vi "Variant-to-String.vi"(11 "Cluster":cluster{"Name":string, "Variant Data":variant}) -> (0 "error out":errorcluster, 3 "String":string)   [LabVIEW 2016, in "SaveLoad.lvlib"]
uses:
  SaveLoad.lvlib
  <vilib>/Utility/Data Type/NI_Data Type.lvlib
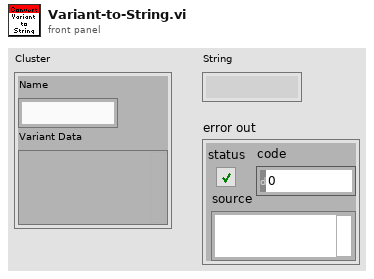
[diagram p1: front panel]
types:
  T1 = typedef "NI_Data Type.lvlib/Data Type.ctl" = enum8{"Invalid Type", "Void", "I8", "I16", "I32", "I64", "U8", "U16", "U32", "U64", "Single Float", "Double Float", "Extended Float", "Single Complex", "Double Complex", "Extended Complex", "Enum U8", "Enum U16", "Enum U32", "Enum U64", "Single Float With Unit", "Double Float With Unit", "Extended Float With Unit", "Single Complex with Unit", "Double Complex with Unit", "Extended Complex with Unit", "Boolean", "String", "Path", "Picture", "Tag", "Array", "Cluster", "Variant", "LV Variant", "Waveform", "Timestamp", "Digital Waveform", "Digital Data", "ExpressData", "Refnum", "External Data", "VI", "Poly VI", "LabVIEW Class Instance", "Fixed Point"}
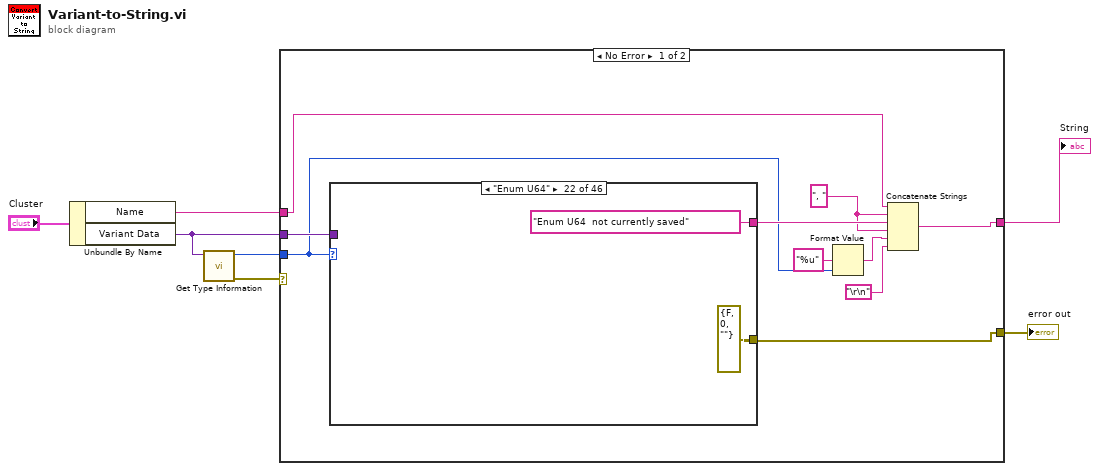
[diagram p0: block diagram]
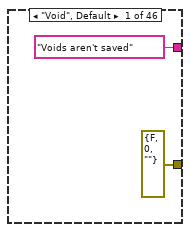
[diagram p2: hidden frame]
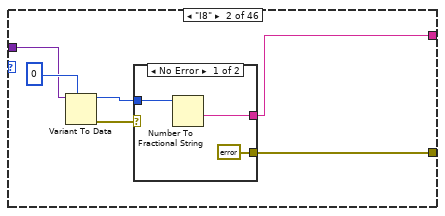
[diagram p3: hidden frame]
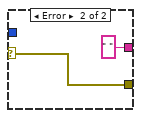
[diagram p4: hidden frame]
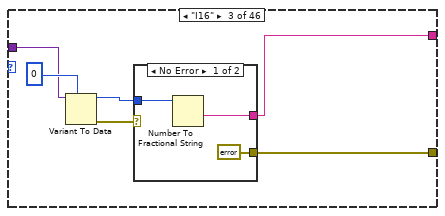
[diagram p5: hidden frame]
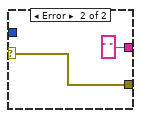
[diagram p6: hidden frame]
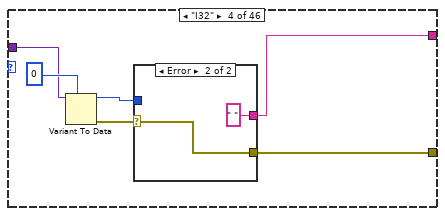
[diagram p7: hidden frame]
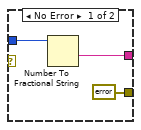
[diagram p8: hidden frame]
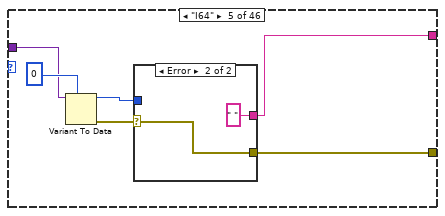
[diagram p9: hidden frame]
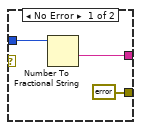
[diagram p10: hidden frame]
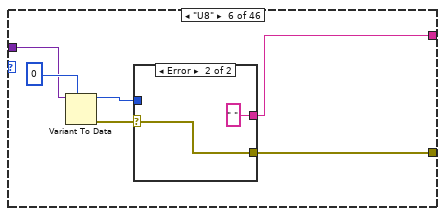
[diagram p11: hidden frame]
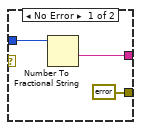
[diagram p12: hidden frame]
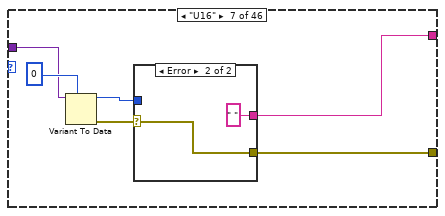
[diagram p13: hidden frame]
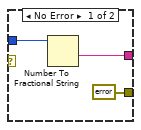
[diagram p14: hidden frame]
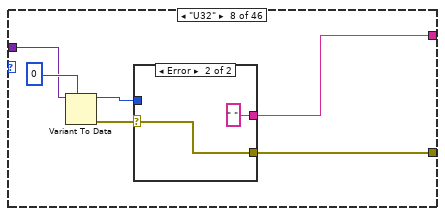
[diagram p15: hidden frame]
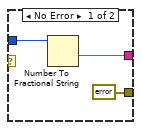
[diagram p16: hidden frame]
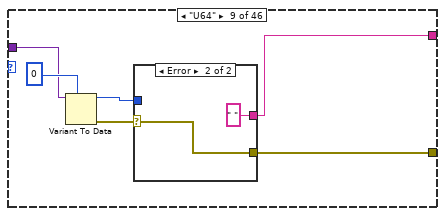
[diagram p17: hidden frame]
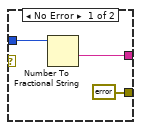
[diagram p18: hidden frame]
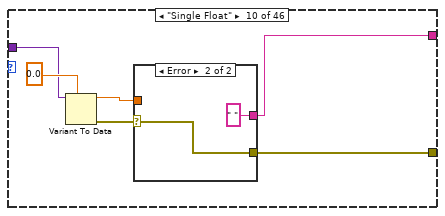
[diagram p19: hidden frame]
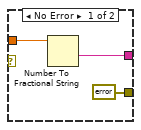
[diagram p20: hidden frame]
diagram:
  n1 = Unbundle By Name("Cluster") -> ("Name"=w5:string, "Variant Data"=w3:variant)
  n2 = call <vilib>:"Get Type Information.vi"("Variant"=w3) -> ("error out"=w1:errorcluster, "Type"=w2:T1)  [unwired: 6 in, 3 out]
  n3 = case shown="No Error" w1 {
    selector: w1 -> [_ w250]
    tunnel: [w15 w250] -> w7
    tunnel: [w16 w247] -> w6
    tunnel: w5 -> [w13 w246]
    tunnel: w3 -> [w17 _]
    tunnel: w2 -> [w10 _]
    frame No Error {
      w11 = ", "
      n4 = case shown="\"Enum U64\"" w10 {
        tunnel: [errorcluster {"status"=FALSE, "code"=0, "source"=""} ("error IO") w21 w32 w43 w53 w65 w76 w87 w98 w109 w120 w131 w142 w154 w164 errorcluster {"status"=FALSE, "code"=0, "source"=""} ("error IO") w177 errorcluster {"status"=FALSE, "code"=0, "source"=""} ("error IO") errorcluster {"status"=FALSE, "code"=0, "source"=""} ("error IO") errorcluster {"status"=FALSE, "code"=0, "source"=""} ("error IO") errorcluster {"status"=FALSE, "code"=0, "source"=""} ("error IO") errorcluster {"status"=FALSE, "code"=0, "source"=""} ("error IO") errorcluster {"status"=FALSE, "code"=0, "source"=""} ("error IO") errorcluster {"status"=FALSE, "code"=0, "source"=""} ("error IO") errorcluster {"status"=FALSE, "code"=0, "source"=""} ("error IO") errorcluster {"status"=FALSE, "code"=0, "source"=""} ("error IO") errorcluster {"status"=FALSE, "code"=0, "source"=""} ("error IO") errorcluster {"status"=FALSE, "code"=0, "source"=""} ("error IO") errorcluster {"status"=FALSE, "code"=0, "source"=""} ("error IO") errorcluster {"status"=FALSE, "code"=0, "source"=""} ("error IO") errorcluster {"status"=FALSE, "code"=0, "source"=""} ("error IO") errorcluster {"status"=FALSE, "code"=0, "source"=""} ("error IO") errorcluster {"status"=FALSE, "code"=0, "source"=""} ("error IO") errorcluster {"status"=FALSE, "code"=0, "source"=""} ("error IO") errorcluster {"status"=FALSE, "code"=0, "source"=""} ("error IO") errorcluster {"status"=FALSE, "code"=0, "source"=""} ("error IO") errorcluster {"status"=FALSE, "code"=0, "source"=""} ("error IO") errorcluster {"status"=FALSE, "code"=0, "source"=""} ("error IO") errorcluster {"status"=FALSE, "code"=0, "source"=""} ("error IO") errorcluster {"status"=FALSE, "code"=0, "source"=""} ("error IO") errorcluster {"status"=FALSE, "code"=0, "source"=""} ("error IO") errorcluster {"status"=FALSE, "code"=0, "source"=""} ("error IO") errorcluster {"status"=FALSE, "code"=0, "source"=""} ("error IO") errorcluster {"status"=FALSE, "code"=0, "source"=""} ("error IO") errorcluster {"status"=FALSE, "code"=0, "source"=""} ("error IO") errorcluster {"status"=FALSE, "code"=0, "source"=""} ("error IO")] -> w15
        tunnel: ["Voids aren't saved" w20 w31 w42 w54 w64 w75 w86 w97 w108 w119 w130 w141 w153 w163 "Clusters not currently saved" w176 "Invalid type" "SGL complex not currently saved" "DBL complex not currently saved" "EXT complex not currently saved" "Enum U64  not currently saved" "Enum U8  not currently saved" "Enum U16  not currently saved" "Enum U32  not currently saved" "SGL w Unit not currently saved" "DBL w Unit not currently saved" "EXT w Unit not currently saved" "SGL complex w Unit not currently saved" "DBL complex w Unit not currently saved" "EXT w Unit not currently saved" "Picture not currently saved" "Tags  not currently saved" "Arrays not currently saved" "Variants not currently saved" "LV Variants not currently saved" "Waveforms not currently saved" "Timestamps  not currently saved" "Digital Waveforms  not currently saved" "Digital data not currently saved" "ExpressData not currently saved" "Refnums not currently saved" "External Data not currently saved" "VIs not currently saved" "Poly VIs not currently saved" "Class Instances not currently saved"] -> w14
        tunnel: w17 -> [_ w23 w34 w45 w56 w67 w78 w89 w100 w111 w122 w133 w144 w156 w166 _ w179 _ _ _ _ _ _ _ _ _ _ _ _ _ _ _ _ _ _ _ _ _ _ _ _ _ _ _ _ _]
        frame "Void", Default {
        }
        frame "I8" {
          n5 = Variant To Data(type=i8 0, Variant=w23) -> (data=w25:i8, error out=w22:errorcluster)  [unwired: 1 in]
          n6 = case shown="No Error" w22 {
            selector: w22 -> [_ w30]
            tunnel: w25 -> [w28 _]
            tunnel: [w27 " "] -> w20
            tunnel: [errorcluster {"status"=FALSE, "code"=0, "source"=""} ("error IO") w30] -> w21
            frame No Error {
              n7 = Number To Fractional String(number=w28) -> (F-format string=w27:string)  [unwired: 3 in]
            }
            frame Error {
            }
          }
        }
        frame "I16" {
          n8 = Variant To Data(type=i16 0, Variant=w34) -> (data=w36:i16, error out=w33:errorcluster)  [unwired: 1 in]
          n9 = case shown="No Error" w33 {
            selector: w33 -> [_ w41]
            tunnel: w36 -> [w39 _]
            tunnel: [w38 " "] -> w31
            tunnel: [errorcluster {"status"=FALSE, "code"=0, "source"=""} ("error IO") w41] -> w32
            frame No Error {
              n10 = Number To Fractional String(number=w39) -> (F-format string=w38:string)  [unwired: 3 in]
            }
            frame Error {
            }
          }
        }
        frame "I32" {
          n11 = Variant To Data(type=0, Variant=w45) -> (data=w47:i32, error out=w44:errorcluster)  [unwired: 1 in]
          n12 = case shown="Error" w44 {
            selector: w44 -> [_ w52]
            tunnel: w47 -> [w50 _]
            tunnel: [w49 " "] -> w42
            tunnel: [errorcluster {"status"=FALSE, "code"=0, "source"=""} ("error IO") w52] -> w43
            frame No Error {
              n13 = Number To Fractional String(number=w50) -> (F-format string=w49:string)  [unwired: 3 in]
            }
            frame Error {
            }
          }
        }
        frame "I64" {
          n14 = Variant To Data(type=i64 0, Variant=w56) -> (data=w58:i64, error out=w55:errorcluster)  [unwired: 1 in]
          n15 = case shown="Error" w55 {
            selector: w55 -> [_ w63]
            tunnel: w58 -> [w61 _]
            tunnel: [w60 " "] -> w54
            tunnel: [errorcluster {"status"=FALSE, "code"=0, "source"=""} ("error IO") w63] -> w53
            frame No Error {
              n16 = Number To Fractional String(number=w61) -> (F-format string=w60:string)  [unwired: 3 in]
            }
            frame Error {
            }
          }
        }
        frame "U8" {
          n17 = Variant To Data(type=u8 0, Variant=w67) -> (data=w69:u8, error out=w66:errorcluster)  [unwired: 1 in]
          n18 = case shown="Error" w66 {
            selector: w66 -> [_ w74]
            tunnel: w69 -> [w72 _]
            tunnel: [w71 " "] -> w64
            tunnel: [errorcluster {"status"=FALSE, "code"=0, "source"=""} ("error IO") w74] -> w65
            frame No Error {
              n19 = Number To Fractional String(number=w72) -> (F-format string=w71:string)  [unwired: 3 in]
            }
            frame Error {
            }
          }
        }
        frame "U16" {
          n20 = Variant To Data(type=u16 0, Variant=w78) -> (data=w80:u16, error out=w77:errorcluster)  [unwired: 1 in]
          n21 = case shown="Error" w77 {
            selector: w77 -> [_ w85]
            tunnel: w80 -> [w83 _]
            tunnel: [w82 " "] -> w75
            tunnel: [errorcluster {"status"=FALSE, "code"=0, "source"=""} ("error IO") w85] -> w76
            frame No Error {
              n22 = Number To Fractional String(number=w83) -> (F-format string=w82:string)  [unwired: 3 in]
            }
            frame Error {
            }
          }
        }
        frame "U32" {
          n23 = Variant To Data(type=u32 0, Variant=w89) -> (data=w91:u32, error out=w88:errorcluster)  [unwired: 1 in]
          n24 = case shown="Error" w88 {
            selector: w88 -> [_ w96]
            tunnel: w91 -> [w94 _]
            tunnel: [w93 " "] -> w86
            tunnel: [errorcluster {"status"=FALSE, "code"=0, "source"=""} ("error IO") w96] -> w87
            frame No Error {
              n25 = Number To Fractional String(number=w94) -> (F-format string=w93:string)  [unwired: 3 in]
            }
            frame Error {
            }
          }
        }
        frame "U64" {
          n26 = Variant To Data(type=u64 0, Variant=w100) -> (data=w102:u64, error out=w99:errorcluster)  [unwired: 1 in]
          n27 = case shown="Error" w99 {
            selector: w99 -> [_ w107]
            tunnel: w102 -> [w105 _]
            tunnel: [w104 " "] -> w97
            tunnel: [errorcluster {"status"=FALSE, "code"=0, "source"=""} ("error IO") w107] -> w98
            frame No Error {
              n28 = Number To Fractional String(number=w105) -> (F-format string=w104:string)  [unwired: 3 in]
            }
            frame Error {
            }
          }
        }
        frame "Single Float" {
          n29 = Variant To Data(type=sgl 0.0, Variant=w111) -> (data=w113:sgl, error out=w110:errorcluster)  [unwired: 1 in]
          n30 = case shown="Error" w110 {
            selector: w110 -> [_ w118]
            tunnel: w113 -> [w116 _]
            tunnel: [w115 " "] -> w108
            tunnel: [errorcluster {"status"=FALSE, "code"=0, "source"=""} ("error IO") w118] -> w109
            frame No Error {
              n31 = Number To Fractional String(number=w116) -> (F-format string=w115:string)  [unwired: 3 in]
            }
            frame Error {
            }
          }
        }
        frame "Double Float" {
          n32 = Variant To Data(type=0.0, Variant=w122) -> (data=w124:dbl, error out=w121:errorcluster)  [unwired: 1 in]
          n33 = case shown="Error" w121 {
            selector: w121 -> [_ w129]
            tunnel: w124 -> [w127 _]
            tunnel: [w126 " "] -> w119
            tunnel: [errorcluster {"status"=FALSE, "code"=0, "source"=""} ("error IO") w129] -> w120
            frame No Error {
              n34 = Number To Fractional String(number=w127) -> (F-format string=w126:string)  [unwired: 3 in]
            }
            frame Error {
            }
          }
        }
        frame "Extended Float" {
          n35 = Variant To Data(type=ext 0.0, Variant=w133) -> (data=w135:ext, error out=w132:errorcluster)  [unwired: 1 in]
          n36 = case shown="Error" w132 {
            selector: w132 -> [_ w140]
            tunnel: w135 -> [w138 _]
            tunnel: [w137 " "] -> w130
            tunnel: [errorcluster {"status"=FALSE, "code"=0, "source"=""} ("error IO") w140] -> w131
            frame No Error {
              n37 = Number To Fractional String(number=w138) -> (F-format string=w137:string)  [unwired: 3 in]
            }
            frame Error {
            }
          }
        }
        frame "Boolean" {
          n38 = Variant To Data(type=FALSE, Variant=w144) -> (data=w146:bool, error out=w143:errorcluster)  [unwired: 1 in]
          n39 = case shown="No Error" w143 {
            selector: w143 -> [_ w152]
            tunnel: w146 -> [w147 _]
            tunnel: [w150 " "] -> w141
            tunnel: [errorcluster {"status"=FALSE, "code"=0, "source"=""} ("error IO") w152] -> w142
            frame No Error {
              n40 = Boolean To (0,1)(Boolean=w147) -> (0, 1=w148:i16)
              n41 = Number To Fractional String(number=w148) -> (F-format string=w150:string)  [unwired: 3 in]
            }
            frame Error {
            }
          }
        }
        frame "String" {
          n42 = Variant To Data(type=" ", Variant=w156) -> (data=w158:string, error out=w155:errorcluster)  [unwired: 1 in]
          n43 = case shown="No Error" w155 {
            selector: w155 -> [_ w162]
            tunnel: w158 -> [w159 _]
            tunnel: [w159 " "] -> w153
            tunnel: [errorcluster {"status"=FALSE, "code"=0, "source"=""} ("error IO") w162] -> w154
            frame No Error {
            }
            frame Error {
            }
          }
        }
        frame "Path" {
          n44 = Variant To Data(type=path "", Variant=w166) -> (data=w168:path, error out=w165:errorcluster)  [unwired: 1 in]
          n45 = case shown="No Error" w165 {
            selector: w165 -> [_ w173]
            tunnel: w168 -> [w171 _]
            tunnel: [w170 " "] -> w163
            tunnel: [errorcluster {"status"=FALSE, "code"=0, "source"=""} ("error IO") w173] -> w164
            frame No Error {
              n46 = Path To String(path=w171) -> (string=w170:string)
            }
            frame Error {
            }
          }
        }
        frame "Cluster" {
        }
        frame "Fixed Point" {
          n47 = Variant To Data(type=fxp<+,1,1> 0.0, Variant=w179) -> (data=w181:fxp<+,1,1>, error out=w178:errorcluster)  [unwired: 1 in]
          n48 = case shown="Error" w178 {
            selector: w178 -> [_ w186]
            tunnel: w181 -> [w184 _]
            tunnel: [w183 " "] -> w176
            tunnel: [errorcluster {"status"=FALSE, "code"=0, "source"=""} ("error IO") w186] -> w177
            frame No Error {
              n49 = Number To Fractional String(number=w184) -> (F-format string=w183:string)  [unwired: 3 in]
            }
            frame Error {
            }
          }
        }
        frame "Invalid Type" {
        }
        frame "Single Complex" {
        }
        frame "Double Complex" {
        }
        frame "Extended Complex" {
        }
        frame "Enum U64" {
        }
        frame "Enum U8" {
        }
        frame "Enum U16" {
        }
        frame "Enum U32" {
        }
        frame "Single Float With Unit" {
        }
        frame "Double Float With Unit" {
        }
        frame "Extended Float With Unit" {
        }
        frame "Single Complex with Unit" {
        }
        frame "Double Complex with Unit" {
        }
        frame "Extended Complex with Unit" {
        }
        frame "Picture" {
        }
        frame "Tag" {
        }
        frame "Array" {
        }
        frame "Variant" {
        }
        frame "LV Variant" {
        }
        frame "Waveform" {
        }
        frame "Timestamp" {
        }
        frame "Digital Waveform" {
        }
        frame "Digital Data" {
        }
        frame "ExpressData" {
        }
        frame "Refnum" {
        }
        frame "External Data" {
        }
        frame "VI" {
        }
        frame "Poly VI" {
        }
        frame "LabVIEW Class Instance" {
        }
      }
      n50 = Format Value(format string="%u", value (0)=w10) -> (output string=w9:string)  [unwired: 1 in]
      n51 = Concatenate Strings(w13, w11, w14, w11, w9, "\r\n") -> (w16:string)
    }
    frame Error {
      n52 = call <vilib>:"Space Constant.vi"() -> ("String"=w245:string)
      n53 = Concatenate Strings(w246, ", ", w245, "\r\n") -> (w247:string)
    }
  }
  "error out" <- w7
  "String" <- w6
